vi "ProcessModbusUpdates.vi"(11 "MockHPILCSettings":T1={"ModbusRxDataFIFO"="MockbusPort2RxFIFO", "ModbusTxDataFIFO"="MockbusPort2TxFIFO", "BufferUpdateFIFO"="MockHPILCCommand", "Code17Memory"="MockHPILCCode17", "Code18Memory"="MockHPILCCode18", "Code65Memory"="MockHPILCCode65", "Code66Memory"="MockHPILCCode66", "Code67Memory"="MockHPILCCode67", "Code72Memory"="MockHPILCCode72", "Code80Memory"="MockHPILCCode80", "Code110Memory"="MockHPILCCode110", "CRCDataFIFO"="MockHPILCCRCDataFIFO", "CRCCalculateFIFO"="MockHPILCCRCCalculateFIFO", "CRCFIFO"="MockHPILCCRCFIFO"}) -> ()   [LabVIEW 2016, in "FPGAMockHPILC.lvlib"]
uses:
  FPGAMockHPILC.lvlib
  DataTypes/MockHPILCSettings.ctl
  DataTypes/MockHPModbusUpdateLoopData.ctl
  DataTypes/MockHPModbusUpdateStates.ctl
  <vilib>/Platform/TimedLoop/XDataNode/timing_clust.ctl
  <vilib>/Platform/TimedLoop/XDataNode/nitl_modes.ctl
  <vilib>/Platform/TimedLoop/XDataNode/wakeup.ctl
  <vilib>/rvi/Emulation/niFpgaSctlEmulationGetInTimedLoop.vi
  <vilib>/rvi/Emulation/niFpgaEmulationReportErrorSimple.vi
  <vilib>/rvi/Emulation/niFpgaGetClockAttributes.vi
  <vilib>/rvi/Emulation/niFpgaCriticalErrorInLSC.vi
  <vilib>/rvi/DataTransferAndStorage/Container/Common/niFpgaContainerExecOnDevCompGetState.vi
  <vilib>/rvi/Emulation/niFpgaEmulationIsFPGAContextNoSignature.vi
  <vilib>/rvi/errors/niFpgaSetErrorForExecOnDevCompSimple.vi
  <vilib>/rvi/eio/common/nirviEmuReportErrorAndStop.vi
  <vilib>/rvi/DataTransferAndStorage/Container/Common/niFpgaContainerGetUniqueNameForEmu.vi
  <vilib>/rvi/FIFO/Fifo_Resource/nirvififoEmulationSetSize.vi
  <vilib>/rvi/FIFO/Fifo_Resource/nirviFifoEmulationQueueMgr.vi
  <instcachedir>/0/nirviFifoEmulationQueueMgr_E5CAEC123FF24DC58D834DCA3CDAA9B5.lvgen/nirviFifoEmulationQueueMgr_E5CAEC123FF24DC58D834DCA3CDAA9B5_002.vi
  <vilib>/rvi/FIFO/Fifo_Resource/nirvififoEmulationDetermineInputValidOut.vi
  <vilib>/rvi/FIFO/Fifo_Resource/nirvififoEmulationCreateLock.vi
  <vilib>/rvi/Emulation/niFpgaProcessEmulError.vi
  <vilib>/rvi/FIFO/Fifo_Resource/nirvififoEmulationObtainLock.vi
  <vilib>/rvi/FIFO/Fifo_Resource/nirvififoEmulationReleaseLock.vi
  <vilib>/rvi/occurrence/nirviWaitOnOccurrenceBase.vi
  <vilib>/rvi/errors/nirviReportUnexpectedCaseInternalError.vi
  <vilib>/rvi/errors/nirviReportUnexpectedCaseInternalError (U32).vi
  <vilib>/Utility/error.llb/Clear Errors.vi
  <vilib>/rvi/interface/RandomDataEmulation/niFpgaRandomDataHandleErrors.vi
  <instcachedir>/0/nirviFifoEmulationQueueMgr_E5CAEC123FF24DC58D834DCA3CDAA9B5.lvgen/nirviFifoEmulationQueueMgr_E5CAEC123FF24DC58D834DCA3CDAA9B5_000.vi
  <vilib>/rvi/Memory/Memory_Emulation/niFpgaMemoryEmulationCacheClearOnFirstRun.vi
  <vilib>/rvi/Memory/Memory_Emulation/nirvimemoryEmulationManagerCache_MakeExclusive.vi
  <vilib>/rvi/Memory/Memory_Emulation/niFpgaMemoryEmulationValidateCache.vi
  <vilib>/rvi/Memory/Memory_Emulation/nirvimemoryEmulationManagerCache_InsertValue.vi
  <vilib>/rvi/Memory/Memory_Emulation/nirvimemoryEmulationManagerCache_ReleaseExclusive.vi
  <vilib>/rvi/Memory/Memory_Emulation/nirvimemoryEmulationManagerCache_GetValue.vi
  <vilib>/rvi/Memory/Memory_Emulation/nirvimemoryEmulationManagerCache_SetValue.vi
  <vilib>/rvi/Emulation/niFpgaSctlEmulationResourceMgr.vi
  <instcachedir>/0/nirviFifoEmulationQueueMgr_E5CAEC123FF24DC58D834DCA3CDAA9B5.lvgen/nirviFifoEmulationQueueMgr_E5CAEC123FF24DC58D834DCA3CDAA9B5_001.vi
  <vilib>/Platform/TimedLoop/XDataNode/XDataNode.xnode
  <vilib>/rvi/DataTransferAndStorage/Container/XNode/niFpgaContainer.xnode
  <vilib>/rvi/FIFO/Fifo_Resource/niFpgaFifoEmulationRefIn.vi
  <vilib>/rvi/Memory/Memory_Emulation/niFpgaMemoryEmulationRefIn.vi
  <vilib>/Platform/TimedLoop/XDataNode/XDNodeRunTimeDep.lvlib
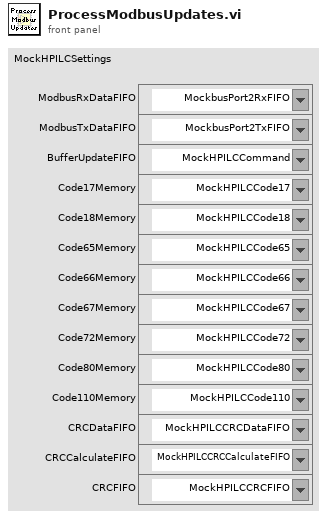
[diagram p1: front panel]
types:
  T1 = typedef "FPGAMockHPILC.lvlib/MockHPILCSettings.ctl" = cluster{"ModbusRxDataFIFO":refnum<k21>, "ModbusTxDataFIFO":refnum<k21>, "BufferUpdateFIFO":refnum<k21>, "Code17Memory":refnum<k21>, "Code18Memory":refnum<k21>, "Code65Memory":refnum<k21>, "Code66Memory":refnum<k21>, "Code67Memory":refnum<k21>, "Code72Memory":refnum<k21>, "Code80Memory":refnum<k21>, "Code110Memory":refnum<k21>, "CRCDataFIFO":refnum<k21>, "CRCCalculateFIFO":refnum<k21>, "CRCFIFO":refnum<k21>}
  T2 = typedef "FPGAMockHPILC.lvlib/MockHPModbusUpdateLoopData.ctl" = cluster{"ModbusUpdateLoopStates":T3, "Address":u8, "Function":u8, "ResponseLength":u8, "ResponseIndex":u8, "Index":u8, "Data":u16, "DelayTicks":u32}
  T3 = typedef "FPGAMockHPILC.lvlib/MockHPModbusUpdateStates.ctl" = enum16{"ReadModbusPort", "ProcessModbusData", "DelayMicroseconds", "WriteAddress", "WriteFunction", "WriteData", "WriteCRCLSB", "WriteCRCMSB", "WriteEndOfFrame", "CalculateCRC"}
  T4 = typedef "XDNodeRunTimeDep.lvlib/timing_clust.ctl" = cluster{"Expected End [f-1]":u64, "Actual End [f-1]":u64, "Finished Late? [f-1]":bool, "Expected End [i-1]":u64, "Actual End [i-1]":u64, "Finished Late? [i-1]":bool, "Expected Start [i]":u64, "Actual Start [i]":u64, "Expected Start [f]":u64, "Actual Start [f]":u64, "Source Name":string, "Structure Name":string, "Period":i64, "Deadline":i64, "Offset":i64, "Start":i64, "Priority":i32, "Timeout":i32, "Mode":T5, "Wakeup Reason":T6, "Error":errorcluster, "Source Type":string, "Secondary Source Type":string, "Global End Time":u64, "Global Start Time":u64, "Frame Duration":u64, "Iteration Duration":u64, "Assigned CPU":i32, "I/O Scan Engine Mode":u32}
  T5 = typedef "XDNodeRunTimeDep.lvlib/nitl_modes.ctl" = enum32{"No Change", "Process missed periods, maintain original phase", "Discard missed periods, maintain original phase", "Process missed periods, ignore original phase", "Discard missed periods, ignore original phase"}
  T6 = typedef "XDNodeRunTimeDep.lvlib/wakeup.ctl" = enum32{"Normal", "Aborted", "Asynchronous wakeup", "Timing source error", "Timed loop error", "Timeout"}
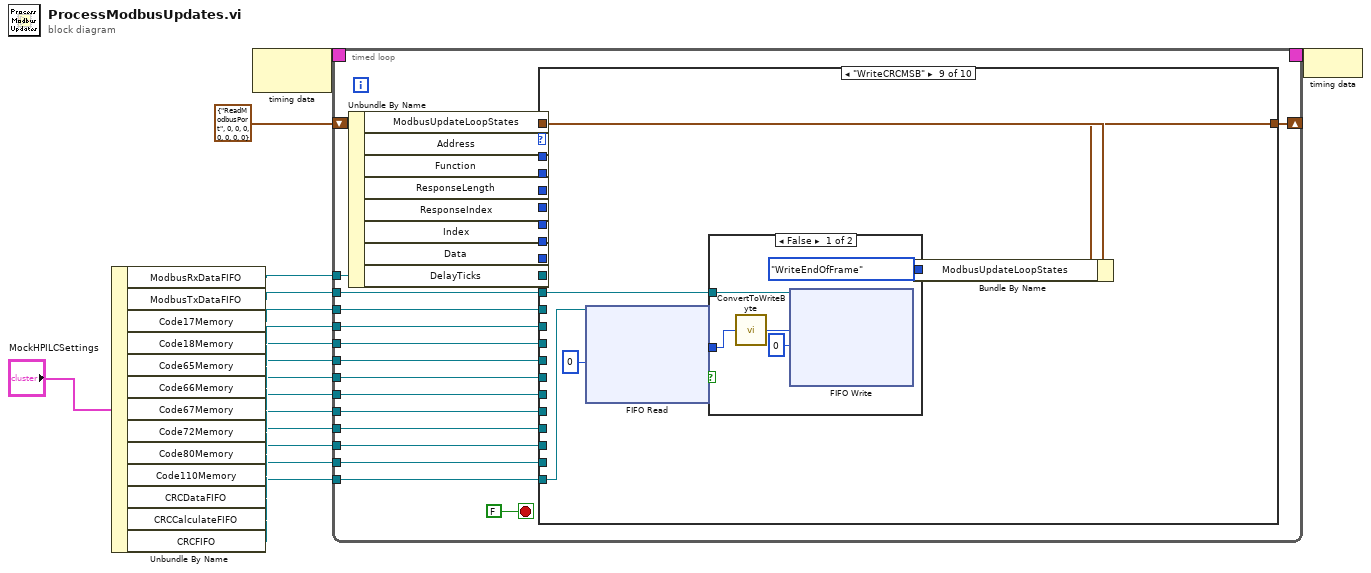
[diagram p0: block diagram]
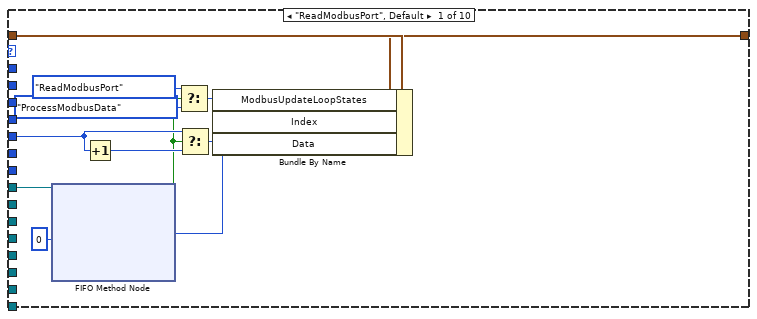
[diagram p2: hidden frame]
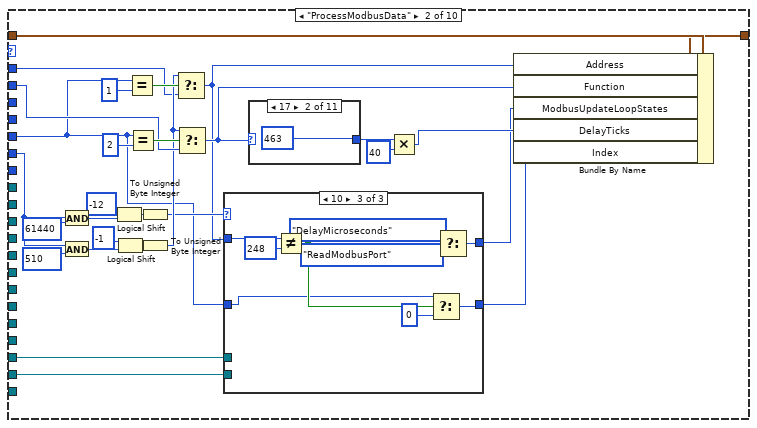
[diagram p3: hidden frame]
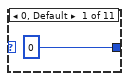
[diagram p4: hidden frame]
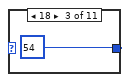
[diagram p5: hidden frame]
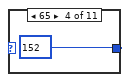
[diagram p6: hidden frame]
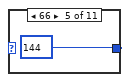
[diagram p7: hidden frame]
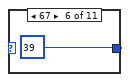
[diagram p8: hidden frame]
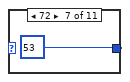
[diagram p9: hidden frame]
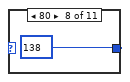
[diagram p10: hidden frame]
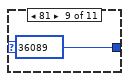
[diagram p11: hidden frame]
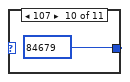
[diagram p12: hidden frame]
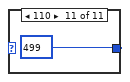
[diagram p13: hidden frame]
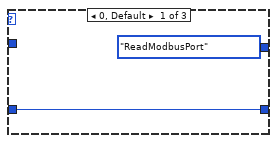
[diagram p14: hidden frame]
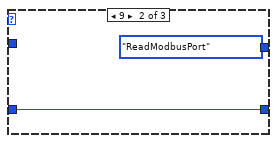
[diagram p15: hidden frame]
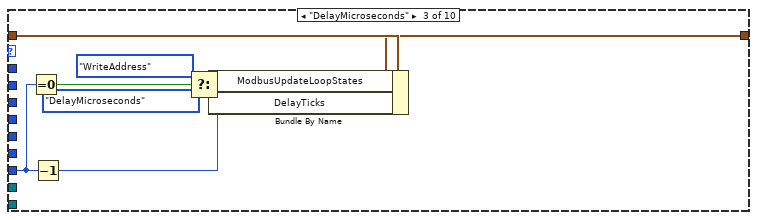
[diagram p16: hidden frame]
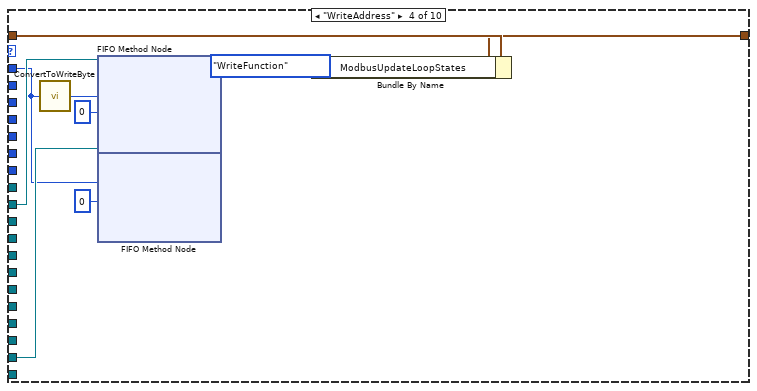
[diagram p17: hidden frame]
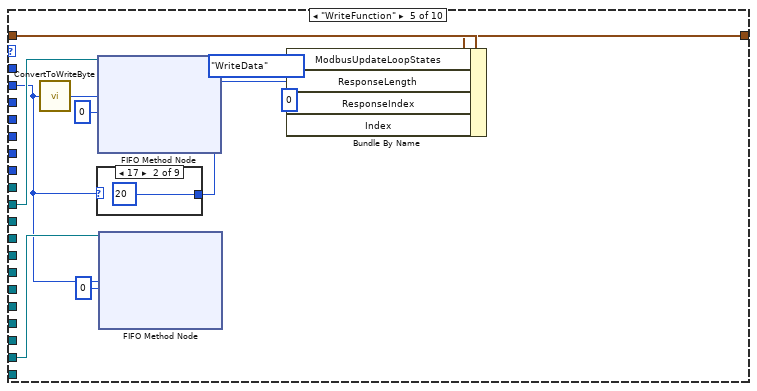
[diagram p18: hidden frame]
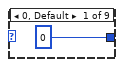
[diagram p19: hidden frame]
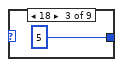
[diagram p20: hidden frame]
diagram:
  n1 = Unbundle By Name("MockHPILCSettings") -> ("ModbusRxDataFIFO"=w13:refnum<k21>, "ModbusTxDataFIFO"=w12:refnum<k21>, "Code17Memory"=w11:refnum<k21>, "Code18Memory"=w10:refnum<k21>, "Code65Memory"=w9:refnum<k21>, "Code66Memory"=w8:refnum<k21>, "Code67Memory"=w7:refnum<k21>, "Code72Memory"=w6:refnum<k21>, "Code80Memory"=w5:refnum<k21>, "Code110Memory"=w4:refnum<k21>, "CRCDataFIFO"=w3:refnum<k21>, "CRCCalculateFIFO"=w2:refnum<k21>, "CRCFIFO"=w1:refnum<k21>)
  n2 = node-c288() -> (w15:T4)  [unwired: 1 in]
  n3 = timed-loop {
    shift-right: [w36] -> _
    shift-left: T2 {"ModbusUpdateLoopStates"=enum."ReadModbusPort", "Address"=0, "Function"=0, "ResponseLength"=0, "ResponseIndex"=0, "Index"=0, "Data"=0, "DelayTicks"=0} ("MockHPBufferUpdateLoopData") -> [w35]
    timing: w15 -> [_]
    timing-out: [_] -> w14
    tunnel: w13 -> [w34]
    tunnel: w12 -> [w30]
    tunnel: w11 -> [w29]
    tunnel: w10 -> [w28]
    tunnel: w9 -> [w27]
    tunnel: w8 -> [w26]
    tunnel: w7 -> [w25]
    tunnel: w6 -> [w24]
    tunnel: w5 -> [w23]
    tunnel: w4 -> [w22]
    tunnel: w3 -> [w18]
    tunnel: w2 -> [w21]
    tunnel: w1 -> [w20]
    stop <- FALSE stop-if-true
    n4 = Unbundle By Name(w35) -> ("ModbusUpdateLoopStates"=w41:T3, "Address"=w40:u8, "Function"=w39:u8, "ResponseLength"=w38:u8, "ResponseIndex"=w37:u8, "Index"=w33:u8, "Data"=w32:u16, "DelayTicks"=w19:u32)
    n5 = case shown="\"WriteCRCMSB\"" w41 {
      tunnel: w40 -> [_ w58 _ w116 _ w168 _ _ _ _]
      tunnel: w39 -> [_ w67 _ _ w125 w171 _ _ _ _]
      tunnel: w38 -> [_ _ _ _ _ w147 _ _ _ _]
      tunnel: w37 -> [_ _ _ _ _ w144 _ _ _ _]
      tunnel: [w44 w81 w113 w118 w129 w172 w223 w234 w248 w256] -> w36
      tunnel: w35 -> [w45 w82 w114 w120 w131 w173 w227 w235 w249 w261]
      tunnel: w34 -> [w53 _ _ _ _ _ _ _ _ _]
      tunnel: w33 -> [w48 w55 _ _ _ _ _ _ _ _]
      tunnel: w32 -> [_ w74 _ _ _ _ _ _ _ _]
      tunnel: w30 -> [_ _ _ w123 w134 w164 _ w229 w243 w260]
      tunnel: w29 -> [_ _ _ _ _ w170 _ _ _ _]
      tunnel: w28 -> [_ _ _ _ _ w163 _ _ _ _]
      tunnel: w27 -> [_ _ _ _ _ w162 _ _ _ _]
      tunnel: w26 -> [_ _ _ _ _ w161 _ _ _ _]
      tunnel: w25 -> [_ _ _ _ _ w160 _ _ _ _]
      tunnel: w24 -> [_ _ _ _ _ w159 _ _ _ _]
      tunnel: w23 -> [_ _ _ _ _ w158 _ _ _ _]
      tunnel: w22 -> [_ _ _ _ _ w157 _ _ _ _]
      tunnel: w18 -> [_ w71 _ w117 w126 w145 _ _ _ _]
      tunnel: w21 -> [_ w70 _ _ _ _ w226 _ _ _]
      tunnel: w20 -> [_ _ _ _ _ _ _ w233 w247 _]
      tunnel: w19 -> [_ _ w108 _ _ _ _ _ _ _]
      frame "ReadModbusPort", Default {
        n6 = xnode ("FIFO Method Node")("Timeout"=0, "FIFO In"=w53) -> ("Element"=w42:u16, "Timed Out?"=w43:bool)  [unwired: 1 out]
        n7 = Increment(x=w48) -> (x+1=w49:u8)
        n8 = Select(t=MockHPModbusUpdateStates."ReadModbusPort", s=w43, f=MockHPModbusUpdateStates."ProcessModbusData") -> (s? t:f=w47:T3)
        n9 = Select(t=w48, s=w43, f=w49) -> (s? t:f=w46:u8)
        n10 = Bundle By Name(cluster=w45, "ModbusUpdateLoopStates"=w47, "Index"=w46, "Data"=w42) -> (w44:T2)
      }
      frame "ProcessModbusData" {
        n11 = And(x=w74, y=u16 61440) -> (x .and. y?=w76:u16)
        n12 = And(x=w74, y=u16 510) -> (x .and. y?=w79:u16)
        n13 = Logical Shift(y=i16 -12, x=w76) -> (x << y=w64:u16)
        n14 = Logical Shift(y=i16 -1, x=w79) -> (x << y=w66:u16)
        n15 = Equal?(x=w55, y=u8 1) -> (x = y?=w72:bool)
        n16 = Equal?(x=w55, y=u8 2) -> (x = y?=w69:bool)
        n17 = To Unsigned Byte Integer(number=w64) -> (unsigned 8bit integer=w63:u8)
        n18 = To Unsigned Byte Integer(number=w66) -> (unsigned 8bit integer=w65:u8)
        n19 = Select(t=w65, s=w72, f=w58) -> (s? t:f=w57:u8)
        n20 = Select(t=w65, s=w69, f=w67) -> (s? t:f=w62:u8)
        n21 = case shown="10" w63 {
          tunnel: w71 -> [_ _ _]
          tunnel: w70 -> [_ _ _]
          tunnel: [MockHPModbusUpdateStates."ReadModbusPort" ("f") MockHPModbusUpdateStates."ReadModbusPort" ("f") w106] -> w56
          tunnel: w57 -> [_ _ w102]
          tunnel: w55 -> [w94 w96 w100]
          tunnel: [w94 w96 w98] -> w54
          frame 0, Default {
          }
          frame 9 {
          }
          frame 10 {
            n22 = Not Equal?(x=w102, y=u8 248) -> (x != y?=w101:bool)
            n23 = Select(t=w100, s=w101, f=u8 0) -> (s? t:f=w98:u8)
            n24 = Select(t=MockHPModbusUpdateStates."DelayMicroseconds" ("f"), s=w101, f=MockHPModbusUpdateStates."ReadModbusPort") -> (s? t:f=w106:T3)
          }
        }
        n25 = case shown="17" w62 {
          tunnel: [u32 0 ("Count(uSec)") u32 463 ("Count(uSec)") u32 54 ("Count(uSec)") u32 152 ("Count(uSec)") u32 144 ("Count(uSec)") u32 39 ("Count(uSec)") u32 53 ("Count(uSec)") u32 138 ("Count(uSec)") u32 36089 ("Count(uSec)") u32 84679 ("Count(uSec)") u32 499 ("Count(uSec)")] -> w61
          frame 0, Default {
          }
          frame 17 {
          }
          frame 18 {
          }
          frame 65 {
          }
          frame 66 {
          }
          frame 67 {
          }
          frame 72 {
          }
          frame 80 {
          }
          frame 81 {
          }
          frame 107 {
          }
          frame 110 {
          }
        }
        n26 = Multiply(x=w61, y=u32 40) -> (x*y=w59:u32)
        n27 = Bundle By Name(cluster=w82, "Address"=w57, "Function"=w62, "ModbusUpdateLoopStates"=w56, "DelayTicks"=w59, "Index"=w54) -> (w81:T2)
      }
      frame "DelayMicroseconds" {
        n28 = Equal To 0?(x=w108) -> (x = 0?=w112:bool)
        n29 = Decrement(x=w108) -> (x-1=w107:u32)
        n30 = Select(t=MockHPModbusUpdateStates."WriteAddress", s=w112, f=MockHPModbusUpdateStates."DelayMicroseconds") -> (s? t:f=w111:T3)
        n31 = Bundle By Name(cluster=w114, "ModbusUpdateLoopStates"=w111, "DelayTicks"=w107) -> (w113:T2)
      }
      frame "WriteAddress" {
        n32 = call "ConvertToWriteByte.vi"("Input"=w116) -> ("Output"=w122:u16)
        n33 = xnode ("FIFO Method Node")("Element"=w122, "Timeout"=0, "FIFO In"=w123) -> ()  [unwired: 2 out]
        n34 = xnode ("FIFO Method Node")("Element"=w116, "Timeout"=0, "FIFO In"=w117) -> ()  [unwired: 2 out]
        n35 = Bundle By Name(cluster=w120, "ModbusUpdateLoopStates"=MockHPModbusUpdateStates."WriteFunction") -> (w118:T2)
      }
      frame "WriteFunction" {
        w127 = u8 0 ("ResponseIndex")
        n36 = call "ConvertToWriteByte.vi"("Input"=w125) -> ("Output"=w133:u16)
        n37 = case shown="17" w125 {
          tunnel: [u8 0 ("ResponseLength") u8 20 ("ResponseLength") u8 5 ("ResponseLength") u8 2 ("ResponseLength") u8 9 ("ResponseLength") u8 9 ("ResponseLength") u8 1 ("ResponseLength") u8 1 ("ResponseLength") u8 96 ("ResponseLength")] -> w128
          frame 0, Default {
          }
          frame 17 {
          }
          frame 18 {
          }
          frame 65 {
          }
          frame 66 {
          }
          frame 67 {
          }
          frame 72 {
          }
          frame 80 {
          }
          frame 110 {
          }
        }
        n38 = xnode ("FIFO Method Node")("Element"=w133, "Timeout"=0, "FIFO In"=w134) -> ()  [unwired: 2 out]
        n39 = xnode ("FIFO Method Node")("Element"=w125, "Timeout"=0, "FIFO In"=w126) -> ()  [unwired: 2 out]
        n40 = Bundle By Name(cluster=w131, "ModbusUpdateLoopStates"=MockHPModbusUpdateStates."WriteData", "ResponseLength"=w128, "ResponseIndex"=w127, "Index"=w127) -> (w129:T2)
      }
      frame "WriteData" {
        n41 = Decrement(x=w168) -> (x-1=w169:u8)
        n42 = Multiply(x=w169, y=w147) -> (x*y=w167:u8)
        n43 = Add(x=w167, y=w144) -> (x+y=w166:u8)
        n44 = case shown="17" w171 {
          tunnel: w170 -> [_ w182 _ _ _ _ _ _ _]
          tunnel: w166 -> [_ w186 w191 w196 w201 w206 w211 w216 w221]
          tunnel: [u8 0 ("Data") w183 w188 w193 w198 w203 w208 w213 w218] -> w165
          tunnel: [FALSE TRUE TRUE TRUE TRUE TRUE TRUE TRUE TRUE] -> w150
          tunnel: w163 -> [_ _ w187 _ _ _ _ _ _]
          tunnel: w162 -> [_ _ _ w192 _ _ _ _ _]
          tunnel: w161 -> [_ _ _ _ w197 _ _ _ _]
          tunnel: w160 -> [_ _ _ _ _ w202 _ _ _]
          tunnel: w159 -> [_ _ _ _ _ _ w207 _ _]
          tunnel: w158 -> [_ _ _ _ _ _ _ w212 _]
          tunnel: w157 -> [_ _ _ _ _ _ _ _ w217]
          frame 0, Default {
          }
          frame 17 {
            n45 = xnode ("Memory Method Node")("Address"=w186, "Memory In"=w182) -> ("Data"=w184:u8)  [unwired: 1 out]
            n46 = feedback-in #1(w184) -> ()
            n47 = feedback #1() -> (w183:u8)  [unwired: 1 in]
          }
          frame 18 {
            n48 = xnode ("Memory Method Node")("Address"=w191, "Memory In"=w187) -> ("Data"=w189:u8)  [unwired: 1 out]
            n49 = feedback-in #2(w189) -> ()
            n50 = feedback #2() -> (w188:u8)  [unwired: 1 in]
          }
          frame 65 {
            n51 = xnode ("Memory Method Node")("Address"=w196, "Memory In"=w192) -> ("Data"=w194:u8)  [unwired: 1 out]
            n52 = feedback-in #3(w194) -> ()
            n53 = feedback #3() -> (w193:u8)  [unwired: 1 in]
          }
          frame 66 {
            n54 = xnode ("Memory Method Node")("Address"=w201, "Memory In"=w197) -> ("Data"=w199:u8)  [unwired: 1 out]
            n55 = feedback-in #4(w199) -> ()
            n56 = feedback #4() -> (w198:u8)  [unwired: 1 in]
          }
          frame 67 {
            n57 = xnode ("Memory Method Node")("Address"=w206, "Memory In"=w202) -> ("Data"=w204:u8)  [unwired: 1 out]
            n58 = feedback-in #5(w204) -> ()
            n59 = feedback #5() -> (w203:u8)  [unwired: 1 in]
          }
          frame 72 {
            n60 = xnode ("Memory Method Node")("Address"=w211, "Memory In"=w207) -> ("Data"=w209:u8)  [unwired: 1 out]
            n61 = feedback-in #6(w209) -> ()
            n62 = feedback #6() -> (w208:u8)  [unwired: 1 in]
          }
          frame 80 {
            n63 = xnode ("Memory Method Node")("Address"=w216, "Memory In"=w212) -> ("Data"=w214:u8)  [unwired: 1 out]
            n64 = feedback-in #7(w214) -> ()
            n65 = feedback #7() -> (w213:u8)  [unwired: 1 in]
          }
          frame 110 {
            n66 = xnode ("Memory Method Node")("Address"=w221, "Memory In"=w217) -> ("Data"=w219:u8)  [unwired: 1 out]
            n67 = feedback-in #8(w219) -> ()
            n68 = feedback #8() -> (w218:u8)  [unwired: 1 in]
          }
        }
        n69 = Increment(x=w144) -> (x+1=w152:u8)
        n70 = Increment(x=w147) -> (x+1=w146:u8)
        n71 = Equal To 0?(x=w144) -> (x = 0?=w151:bool)
        n72 = Equal?(x=w146, y=w152) -> (x = y?=w156:bool)
        n73 = Select(t=FALSE, s=w151, f=w150) -> (s? t:f=w149:bool)
        n74 = case shown="True" w149 {
          tunnel: w165 -> [_ w175]
          tunnel: w164 -> [_ w177]
          tunnel: w145 -> [_ w176]
          frame False {
          }
          frame True {
            n75 = call "ConvertToWriteByte.vi"("Input"=w175) -> ("Output"=w178:u16)
            n76 = xnode ("FIFO Method Node")("Element"=w178, "Timeout"=0, "FIFO In"=w177) -> ()  [unwired: 2 out]
            n77 = xnode ("FIFO Method Node")("Element"=w175, "Timeout"=0, "FIFO In"=w176) -> ()  [unwired: 2 out]
          }
        }
        n78 = Select(t=MockHPModbusUpdateStates."CalculateCRC", s=w156, f=MockHPModbusUpdateStates."WriteData") -> (s? t:f=w153:T3)
        n79 = Bundle By Name(cluster=w173, "ModbusUpdateLoopStates"=w153, "ResponseIndex"=w152) -> (w172:T2)
      }
      frame "CalculateCRC" {
        n80 = xnode ("FIFO Write")("Element"=TRUE, "Timeout"=0, "FIFO In"=w226) -> ()  [unwired: 2 out]
        n81 = Bundle By Name(cluster=w227, "ModbusUpdateLoopStates"=MockHPModbusUpdateStates."WriteCRCLSB") -> (w223:T2)
      }
      frame "WriteCRCLSB" {
        n82 = xnode ("FIFO Read")("Timeout"=0, "FIFO In"=w233) -> ("Element"=w230:u8, "Timed Out?"=w231:bool)  [unwired: 1 out]
        n83 = case shown="False" w231 {
          tunnel: w230 -> [w240 _]
          tunnel: w229 -> [w239 _]
          tunnel: [MockHPModbusUpdateStates."WriteCRCMSB" ("ModbusUpdateLoopStates") MockHPModbusUpdateStates."WriteCRCLSB" ("ModbusUpdateLoopStates")] -> w228
          frame False {
            n84 = call "ConvertToWriteByte.vi"("Input"=w240) -> ("Output"=w238:u16)
            n85 = xnode ("FIFO Write")("Element"=w238, "Timeout"=0, "FIFO In"=w239) -> ()  [unwired: 2 out]
          }
          frame True {
          }
        }
        n86 = Bundle By Name(cluster=w235, "ModbusUpdateLoopStates"=w228) -> (w234:T2)
      }
      frame "WriteCRCMSB" {
        n87 = xnode ("FIFO Read")("Timeout"=0, "FIFO In"=w247) -> ("Element"=w244:u8, "Timed Out?"=w245:bool)  [unwired: 1 out]
        n88 = case shown="False" w245 {
          tunnel: w244 -> [w254 _]
          tunnel: w243 -> [w253 _]
          tunnel: [MockHPModbusUpdateStates."WriteEndOfFrame" ("ModbusUpdateLoopStates") MockHPModbusUpdateStates."WriteCRCMSB" ("ModbusUpdateLoopStates")] -> w242
          frame False {
            n89 = call "ConvertToWriteByte.vi"("Input"=w254) -> ("Output"=w252:u16)
            n90 = xnode ("FIFO Write")("Element"=w252, "Timeout"=0, "FIFO In"=w253) -> ()  [unwired: 2 out]
          }
          frame True {
          }
        }
        n91 = Bundle By Name(cluster=w249, "ModbusUpdateLoopStates"=w242) -> (w248:T2)
      }
      frame "WriteEndOfFrame" {
        n92 = xnode ("FIFO Write")("Element"=u16 8416, "Timeout"=0, "FIFO In"=w260) -> ()  [unwired: 2 out]
        n93 = Bundle By Name(cluster=w261, "ModbusUpdateLoopStates"=MockHPModbusUpdateStates."ReadModbusPort") -> (w256:T2)
      }
    }
  }
  n94 = node-c288(w14) -> ()
